vi "Main.vi"() -> ()   [LabVIEW 2017]
uses:
  TypeDefs/command.ctl
  TypeDefs/Admittance Coefficients.ctl
  TypeDefs/allData.ctl
  TypeDefs/coord.ctl
panel:
  in  "Admittance Coeffs":T1
  in  "Velocity (mm/s)":dbl
  in  "Attractor point":T2
  in  "Target Point":T2
  in  "Start Point":T2
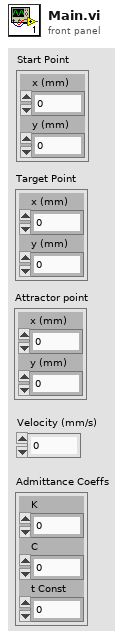
[diagram p1: front panel]
types:
  T1 = typedef "Admittance Coefficients.ctl" = cluster{"K":dbl, "C":dbl, "t Const":dbl}
  T2 = typedef "coord.ctl" = cluster{"x (mm)":dbl, "y (mm)":dbl}
  T3 = typedef "allData.ctl" = cluster{"xi":dbl, "yi":dbl, "xf":dbl, "yf":dbl, "tf":dbl, "xlamda":dbl, "ylamda":dbl, "xt":dbl, "yt":dbl, "Admittance Coeffs":T1}
  T4 = typedef "command.ctl" = enum16{"end", "run", "init"}
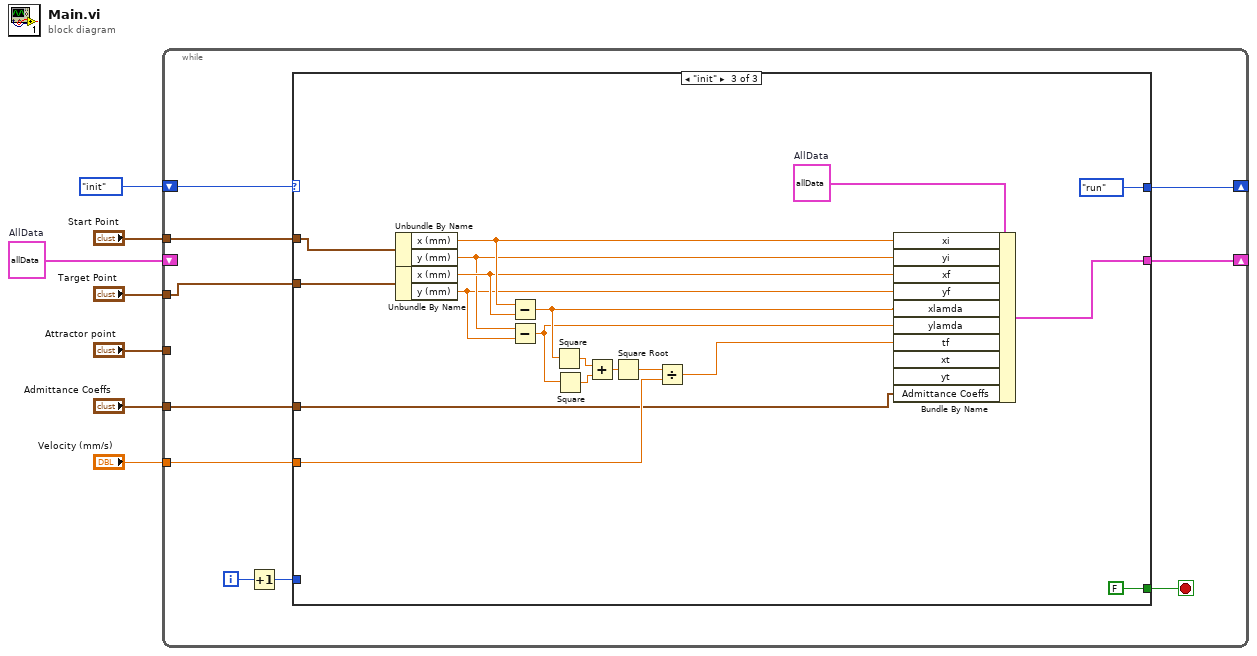
[diagram p0: block diagram]
diagram:
  w1 = T3 {"xi"=0.0, "yi"=0.0, "xf"=0.0, "yf"=0.0, "tf"=0.0, "xlamda"=0.0, "ylamda"=0.0, "xt"=0.0, "yt"=0.0, "Admittance Coeffs"={"K"=0.0, "C"=0.0, "t Const"=0.0}}  # AllData
  n1 = while {
    shift-right: [w16] -> _
    shift-left: command."init" -> [w17]
    tunnel: "Start Point" -> [w13]
    tunnel: "Target Point" -> [w12]
    tunnel: "Attractor point" -> [_]
    tunnel: "Admittance Coeffs" -> [w8]
    tunnel: "Velocity (mm/s)" -> [w11]
    shift-right: [w14] -> _
    shift-left: w1 -> [_]
    i -> [w10]
    stop <- w15 stop-if-true
    n2 = Increment(x=w10) -> (x+1=w9:i32)
    n3 = case shown="\"init\"" w17 {
      tunnel: [_ _ command."run"] -> w16
      tunnel: [_ _ FALSE] -> w15
      tunnel: [_ _ w33] -> w14
      tunnel: w13 -> [_ _ w32]
      tunnel: w12 -> [_ _ w31]
      tunnel: w11 -> [_ _ w22]
      tunnel: w9 -> [_ _ _]
      tunnel: w8 -> [_ _ w18]
      frame "end", Default {
      }
      frame "run" {
      }
      frame "init" {
        w36 = T3 {"xi"=0.0, "yi"=0.0, "xf"=0.0, "yf"=0.0, "tf"=0.0, "xlamda"=0.0, "ylamda"=0.0, "xt"=0.0, "yt"=0.0, "Admittance Coeffs"={"K"=0.0, "C"=0.0, "t Const"=0.0}}  # AllData
        n4 = Unbundle By Name(w32) -> ("x (mm)"=w30:dbl, "y (mm)"=w28:dbl)
        n5 = Unbundle By Name(w31) -> ("x (mm)"=w29:dbl, "y (mm)"=w27:dbl)
        n6 = Subtract(x=w30, y=w29) -> (x-y=w20:dbl)
        n7 = Subtract(x=w28, y=w27) -> (x-y=w19:dbl)
        n8 = Square(x=w20) -> (x^2=w25:dbl)
        n9 = Square(x=w19) -> (x^2=w26:dbl)
        n10 = Add(x=w25, y=w26) -> (x+y=w24:dbl)
        n11 = Square Root(x=w24) -> (sqrt(x)=w23:dbl)
        n12 = Divide(x=w23, y=w22) -> (x/y=w21:dbl)
        n13 = Bundle By Name(cluster=w36, "xi"=w30, "yi"=w28, "xf"=w29, "yf"=w27, "xlamda"=w20, "ylamda"=w19, "tf"=w21, "Admittance Coeffs"=w18) -> (w33:T3)  [unwired: 2 in]
      }
    }
  }
